vi "UTILITY Robocopy.vi"(6 "Refresh Programs Named":string, 7 "Robocopy Status":enum16{"Enable", "Disable"}(ring), 8 "Error In":errorcluster, 9 "Previous Hour":i32, 10 "Save Every x Hour":i32=2, 11 "Robocopy Location Command":string) -> (0 "Error Out":errorcluster, 2 "Hour":i32, 3 "Push Data":bool)   [LabVIEW 2014]
panel:
  out "date/time string":string
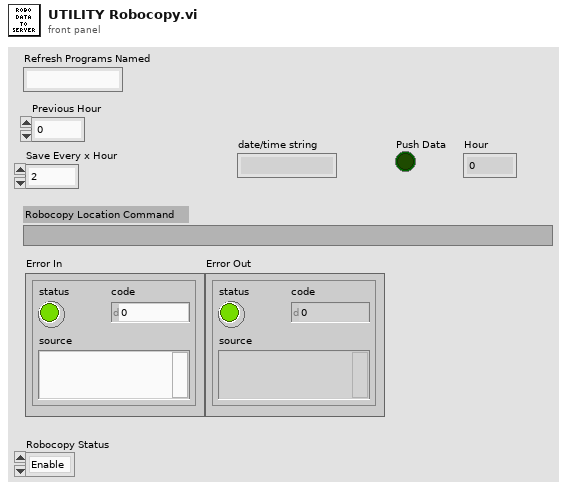
[diagram p1: front panel]
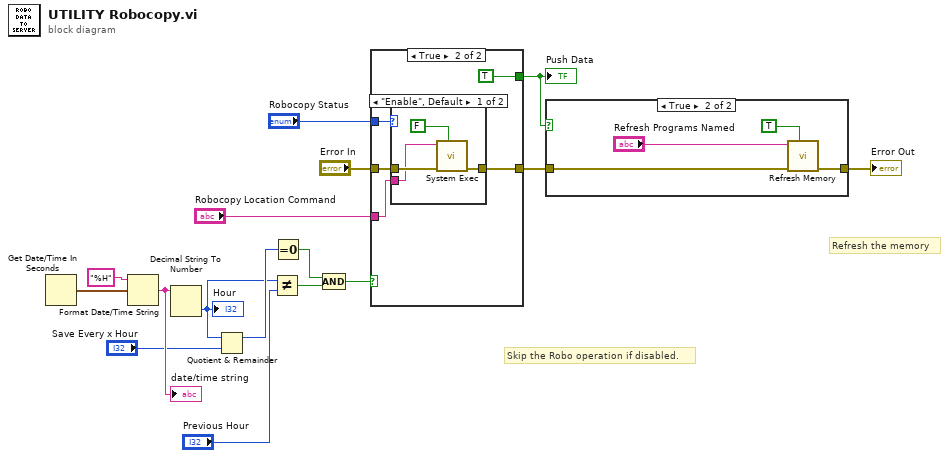
[diagram p0: block diagram]
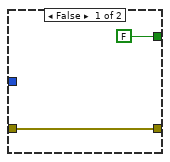
[diagram p3: hidden frame]
diagram:
  # "Refresh the memory"
  # "Skip the Robo operation if disabled."
  n1 = Get Date/Time In Seconds() -> (seconds since 1Jan1904=w16:timestamp)
  n2 = Format Date/Time String(time format string (%c)="%H", seconds (now)=w16) -> (date/time string=w14:string)  [unwired: 1 in]
  "date/time string" <- w14
  n3 = Decimal String To Number(string=w14) -> (number=w9:i32)  [unwired: 2 in, 1 out]
  "Hour" <- w9
  n4 = Quotient & Remainder(x=w9, y="Save Every x Hour") -> (x-y*floor(x/y)=w12:i32)  [unwired: 1 out]
  n5 = Not Equal?(x=w9, y="Previous Hour") -> (x != y?=w6:bool)
  n6 = Equal To 0?(x=w12) -> (x = 0?=w7:bool)
  n7 = Compound Arithmetic op=AND(w7, w6) -> (w5:bool)
  n8 = case shown="True" w5 {
    tunnel: "Error In" -> [w18 w23]
    tunnel: [w18 w22] -> w2
    tunnel: "Robocopy Location Command" -> [_ w21]
    tunnel: [FALSE TRUE] -> w3
    tunnel: "Robocopy Status" -> [_ w19]
    frame False {
    }
    frame True {
      n9 = case shown="\"Enable\", Default" w19 {
        tunnel: w23 -> [w27 w28]
        tunnel: [w26 w28] -> w22
        tunnel: w21 -> [w25 _]
        frame "Enable", Default {
          n10 = call <vilib>:"System Exec.vi"("wait until completion? (T)"=FALSE, "error in (no error)"=w27, "command line"=w25) -> ("error out"=w26:errorcluster)  [unwired: 5 in, 3 out]
        }
        frame "Disable" {
        }
      }
    }
  }
  "Push Data" <- w3
  n11 = case shown="True" w3 {
    tunnel: w2 -> [w29 w31]
    tunnel: [w29 w30] -> w1
    frame False {
    }
    frame True {
      n12 = call "Refresh Memory.vi"("Refresh?"=TRUE, "Error In"=w31, "Refresh Programs Named"="Refresh Programs Named") -> ("Error Out"=w30:errorcluster)  [unwired: 7 in, 1 out]
    }
  }
  "Error Out" <- w1
